vi "Safe Hardware.vi"(8 "error in (no error)":errorcluster, 11 "Process Settings in":refnum<class "Process Settings.lvclass">) -> (0 "error out":errorcluster, 3 "Process Settings out":refnum<class "Process Settings.lvclass">)   [LabVIEW 2017, in "Saturation.lvclass"]
uses:
  Saturation.lvclass
  Process Settings/Process Settings.lvclass
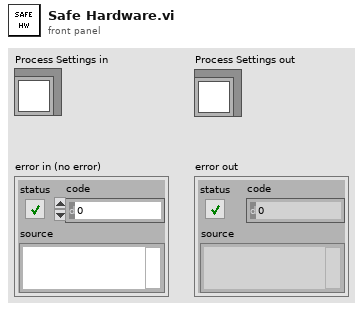
[diagram p1: front panel]
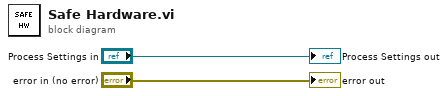
[diagram p0: block diagram]
diagram:
  "Process Settings out" <- "Process Settings in"
  "error out" <- "error in (no error)"
